vi "Set Device Baud Rate.vi"(8 "Error In":errorcluster, 10 "Baud Rate":u32, 11 "LINX Device Config":T1) -> (0 "Error Out":errorcluster, 2 "Baud Rate":u32, 3 "LINX Device Config":T1)   [LabVIEW 2011, in "LVH-LINX.lvlib" / "Device.lvlib"]
uses:
  Device.lvlib
  Type Defs/LINX Device Config.ctl
  Type Defs/Interface.ctl
  Type Defs/TCP Config.ctl
  Type Defs/Error Type.ctl
  LVH-LINX.lvlib
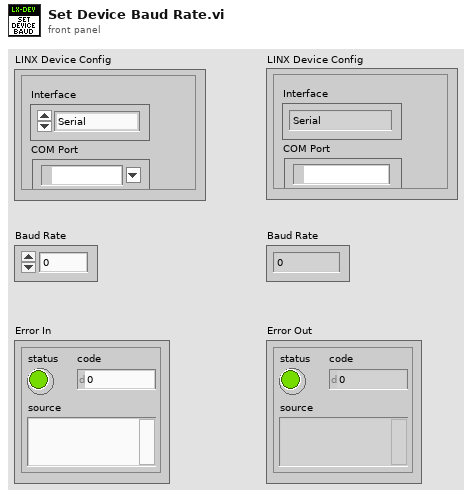
[diagram p1: front panel]
types:
  T1 = typedef "LVH-LINX.lvlib/LINX Device Config.ctl" = cluster{"Interface":T2, "COM Port":refnum<visa-resource-name>, "Packet Number":u16, "TCP Configuration":T3, "Device Family":u8, "Device ID":u8, "Device Name":string}
  T2 = typedef "LVH-LINX.lvlib/Interface.ctl" = enum16{"Serial", "TCP"}
  T3 = typedef "LVH-LINX.lvlib/TCP Config.ctl" = cluster{"IP Address":string, "Port":dbl}
  T4 = typedef "LVH-LINX.lvlib/Error Type.ctl" = enum16{"Unknown", "Timeout", "Corrupt Return Packet", "Unable To Connect", "Command Not Supported"}
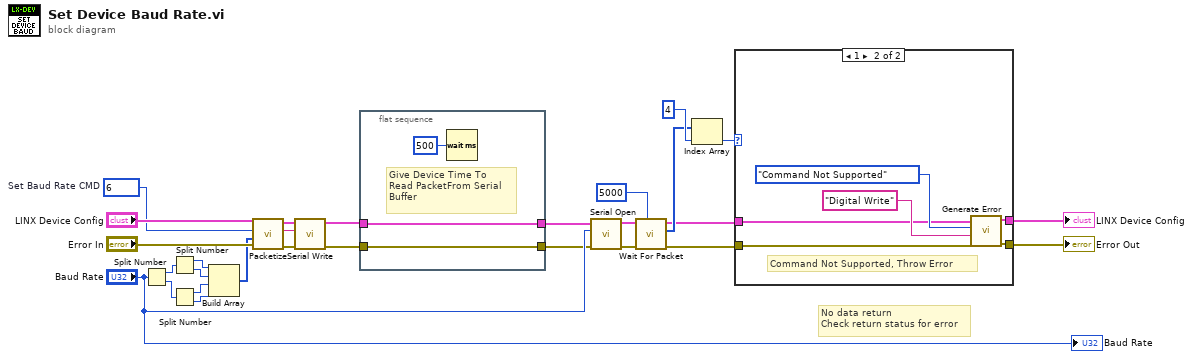
[diagram p0: block diagram]
diagram:
  w15 = u16 6  # Set Baud Rate CMD
  # "No data return\nCheck return status for error"
  n1 = Split Number(x="Baud Rate") -> (hi(x)=w24:u16, lo(x)=w25:u16)
  n2 = Split Number(x=w24) -> (hi(x)=w23:u8, lo(x)=w22:u8)
  n3 = Split Number(x=w25) -> (hi(x)=w21:u8, lo(x)=w20:u8)
  n4 = Build Array(w23, w22, w21, w20) -> (w14:u8[])
  n5 = call "Packetize.vi"("Error In"="Error In", "ARGS"=w14, "CMD"=w15, "LINX Device Config"="LINX Device Config") -> ("Error Out"=w18:errorcluster, "Packet"=w5:string, "LINX Decice Config"=w19:T1)  [unwired: 5 in]
  n6 = call "Serial Write.vi"("Error In"=w18, "Data"=w5, "LINX Device Config"=w19) -> ("Error Out"=w3:errorcluster, "LINX Device Config"=w2:T1)  [unwired: 7 in]
  n7 = flat-sequence {
    tunnel: [w30] -> w4
    tunnel: w3 -> [w30]
    tunnel: w2 -> [w29]
    tunnel: [w29] -> w1
    frame #0 {
      # "Give Device Time To \nRead PacketFrom Serial \nBuffer"
      n8 = Wait (ms)(milliseconds to wait=u32 500) -> ()  [unwired: 1 out]
    }
  }
  n9 = call "Serial Open.vi"("Error In"=w4, "Baud Rate"="Baud Rate", "LINX Device Config"=w1) -> ("Error Out"=w7:errorcluster, "LINX Device Config"=w8:T1)  [unwired: 7 in]
  n10 = call "Wait For Packet.vi"("Timeout (100 ms)"=u32 5000, "Error In"=w7, "LINX Device Config"=w8) -> ("Error Out"=w11:errorcluster, "Packet"=w12:u8[], "LINX Device Config"=w9:T1)  [unwired: 6 in]
  n11 = Index Array(array=w12, index=4) -> (element=w13:u8)
  n12 = case shown="1" w13 {
    tunnel: [w33 w38] -> w27
    tunnel: [w32 w39] -> w26
    tunnel: w11 -> [w32 w35]
    tunnel: w9 -> [w33 w34]
    frame 0, Default {
      # "Read Device Reboot Delay"
      # "Status OK"
    }
    frame 1 {
      # "Command Not Supported, Throw Error"
      n13 = call "Generate Error.vi"("Error In"=w35, "Arguments"="Digital Write", "Error Type"=Error_Type."Command Not Supported", "LINX Device Config"=w34) -> ("Error Out"=w39:errorcluster, "LINX Device Config"=w38:T1)  [unwired: 6 in]
    }
  }
  "Error Out" <- w26
  "LINX Device Config" <- w27
  "Baud Rate" <- "Baud Rate"
